vi "byte test.vi"() -> ()   [LabVIEW 2024]
uses:
  <vilib>/Instr/_visa.llb/VISA Configure Serial Port (Instr).vi
panel:
  in  "Boolean":bool
  in  "number 2":dbl[](array[numeric])
  in  "Enum":enum16{"write", "Read"}(ring)
  in  "number":dbl[](array[numeric])
  in  "VISA resource name 2":refnum<visa-resource-name>
  out "error out 2":errorcluster
  out "unsigned byte array":u8[](array[numeric])
  in  "VISA resource name":refnum<visa-resource-name>
  out "error out":errorcluster
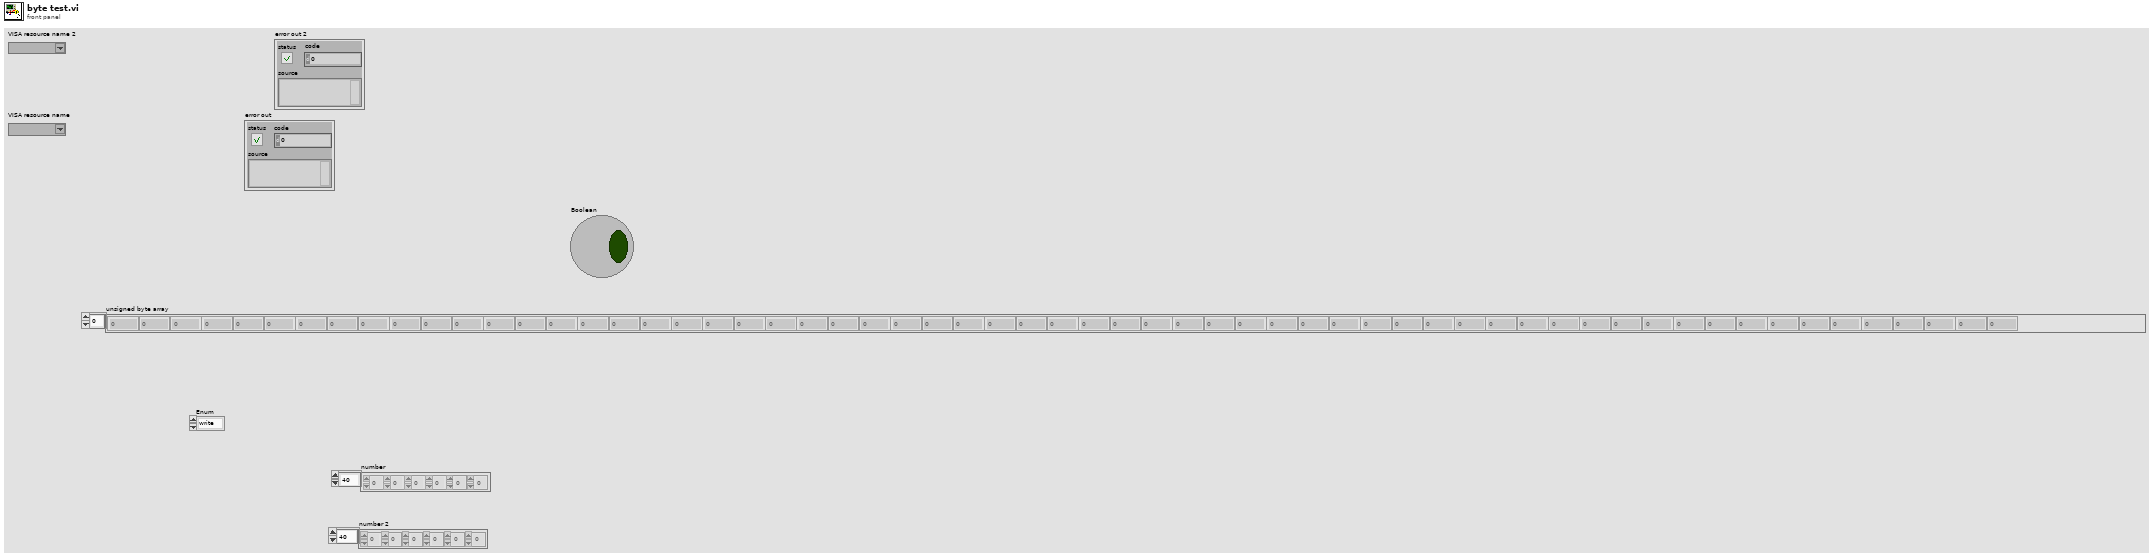
[diagram p1: front panel]
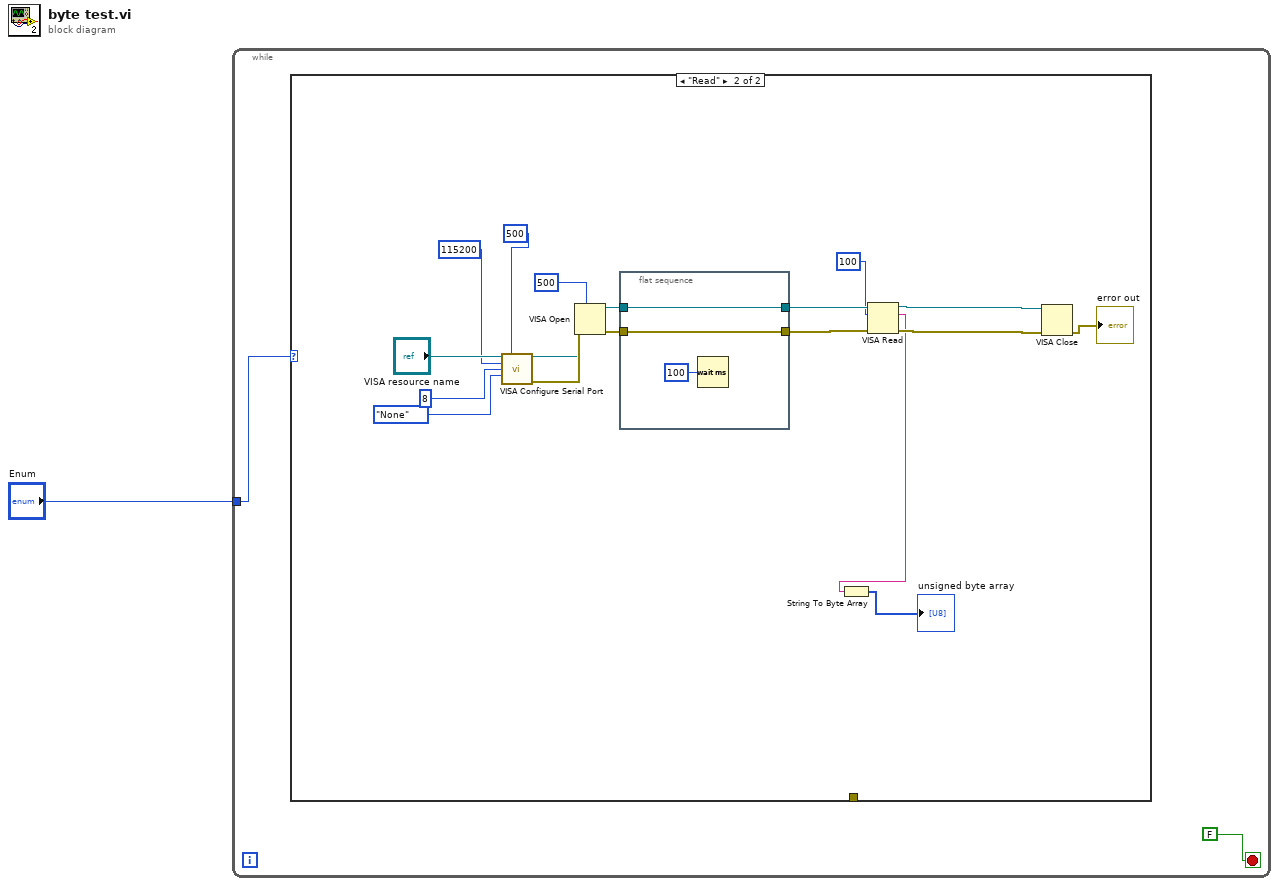
[diagram p0: block diagram]
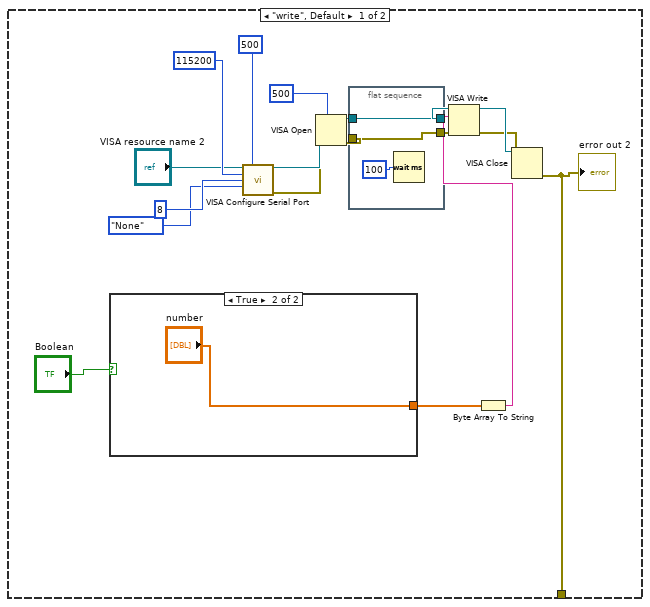
[diagram p2: hidden frame]
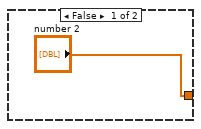
[diagram p3: hidden frame]
diagram:
  n1 = while {
    tunnel: "Enum" -> [w3]
    stop <- FALSE stop-if-true
    n2 = case shown="\"Read\"" w3 {
      tunnel: [w8 _] -> _
      frame "write", Default {
        n3 = case shown="True" "Boolean" {
          tunnel: ["number 2" "number"] -> w11
          frame False {
          }
          frame True {
          }
        }
        n4 = call-poly "VISA Configure Serial Port"("VISA resource name"="VISA resource name 2", "timeout (10sec)"=u32 500, "baud rate (9600)"=u32 115200, "data bits (8)"=u16 8, "parity (0:none)"=enum16{"None", "Odd", "Even", "Mark", "Space"}."None") -> ("VISA resource name out"=w19:refnum<visa-resource-name>, "error out"=w18:errorcluster)  [unwired: 9 in]
        n5 = VISA Open(timeout (0)=u32 500 ("VISA Open timeout (0)"), error in (no error)=w18, VISA resource name=w19) -> (VISA resource name=w5:refnum<visa-resource-name>, error out=w6:errorcluster)  [unwired: 2 in]
        n6 = flat-sequence {
          tunnel: [w24] -> w7
          tunnel: w6 -> [w24]
          tunnel: w5 -> [w23]
          tunnel: [w23] -> w4
          frame #0 {
            n7 = Wait (ms)(milliseconds to wait=u32 100) -> ()  [unwired: 1 out]
          }
        }
        n8 = Byte Array To String(unsigned byte array=w11) -> (string=w10:string)
        n9 = VISA Write(VISA resource name=w4, write buffer=w10, error in (no error)=w7) -> (VISA resource name out=w13:refnum<visa-resource-name>, error out=w12:errorcluster)  [unwired: 1 out]
        n10 = VISA Close(VISA resource name=w13, error in (no error)=w12) -> (error out=w8:errorcluster)
        "error out 2" <- w8
      }
      frame "Read" {
        n11 = call-poly "VISA Configure Serial Port"("VISA resource name"="VISA resource name", "timeout (10sec)"=u32 500, "baud rate (9600)"=u32 115200, "data bits (8)"=u16 8, "parity (0:none)"=enum16{"None", "Odd", "Even", "Mark", "Space"}."None") -> ("VISA resource name out"=w40:refnum<visa-resource-name>, "error out"=w41:errorcluster)  [unwired: 9 in]
        n12 = VISA Open(timeout (0)=u32 500 ("VISA Open timeout (0)"), error in (no error)=w41, VISA resource name=w40) -> (VISA resource name=w33:refnum<visa-resource-name>, error out=w31:errorcluster)  [unwired: 2 in]
        n13 = flat-sequence {
          tunnel: w33 -> [w47]
          tunnel: [w47] -> w32
          tunnel: w31 -> [w46]
          tunnel: [w46] -> w30
          frame #0 {
            n14 = Wait (ms)(milliseconds to wait=u32 100) -> ()  [unwired: 1 out]
          }
        }
        n15 = VISA Read(VISA resource name=w32, byte count=u32 100, error in (no error)=w30) -> (VISA resource name out=w42:refnum<visa-resource-name>, read buffer=w29:string, error out=w43:errorcluster)  [unwired: 1 out]
        n16 = String To Byte Array(string=w29) -> (unsigned byte array=→"unsigned byte array":u8[])
        n17 = VISA Close(VISA resource name=w42, error in (no error)=w43) -> (error out=→"error out":errorcluster)
      }
    }
  }
